vi "uDAQreadData.vi"(4 "Data Header":u8[](array[numeric])=[0, 255, 0], 5 "Process":string, 6 "DataStart":i32, 7 "Residual Buffer in":string[](array[string])=["", "", "", "", "", "", "", ""], 9 "ByteArray":u8[](array[numeric])=array[5000 elements], 10 "FS Range":sgl, 11 "NextArrayBuf":i32) -> (1 "Data":dbl[](array[numeric]), 3 "Residual Buffer out":string[](array[string]))   [LabVIEW 2017]
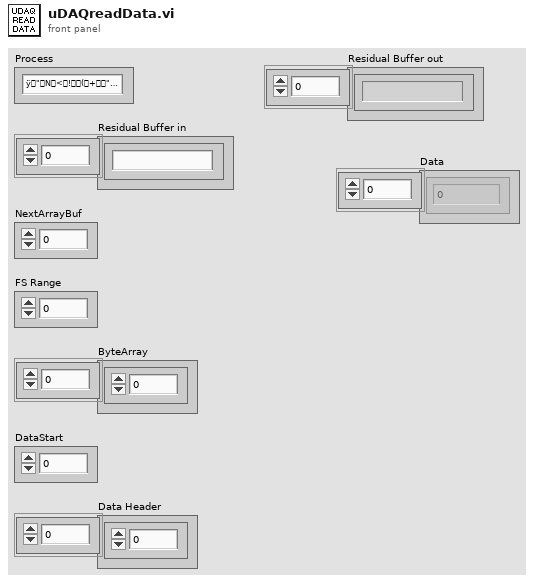
[diagram p1: front panel]
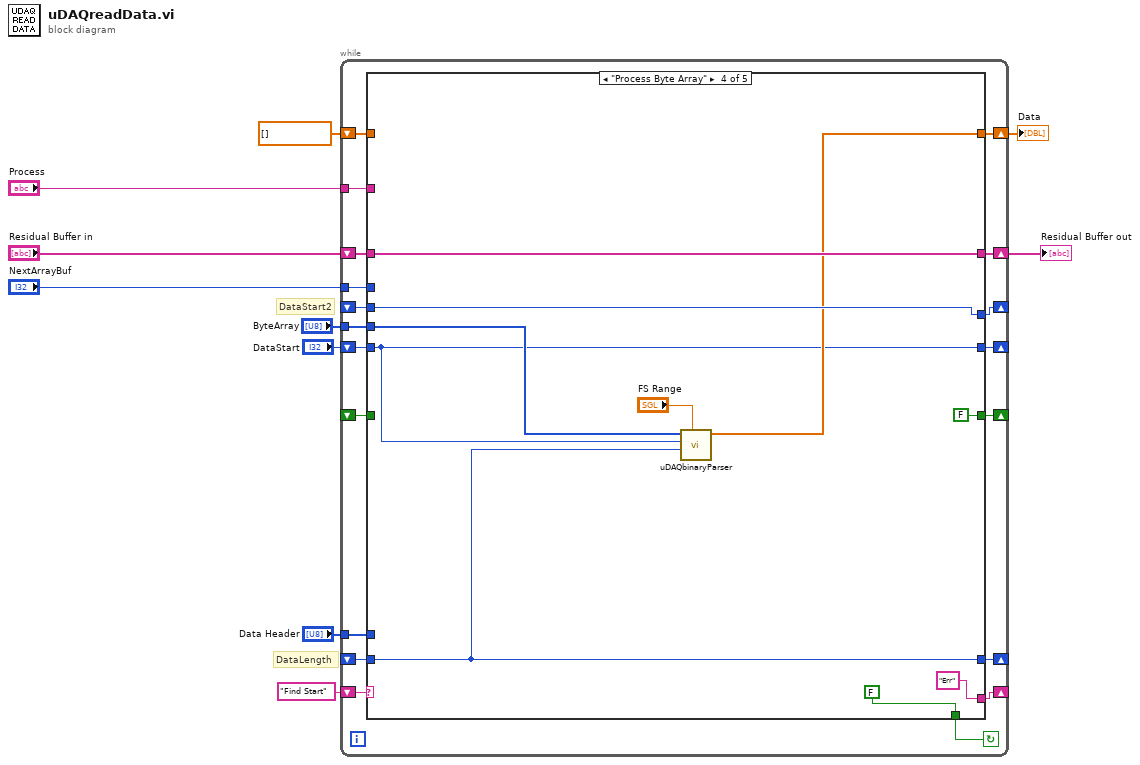
[diagram p0: block diagram]
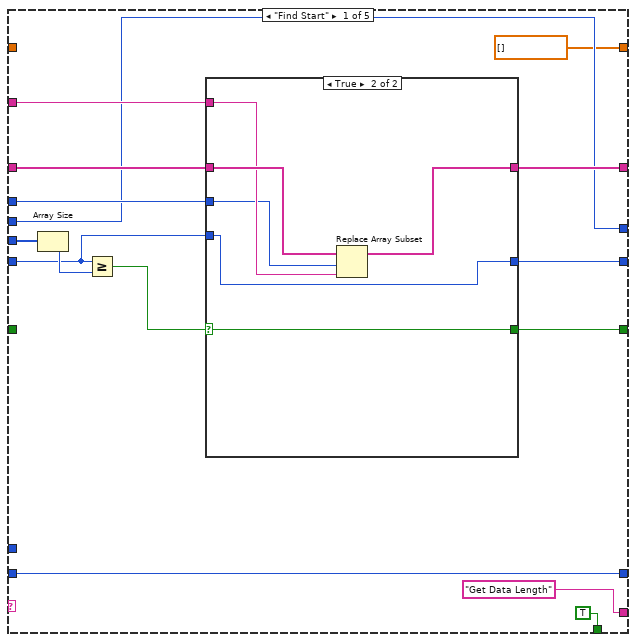
[diagram p2: hidden frame]
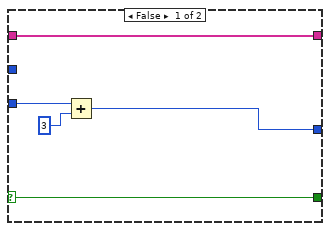
[diagram p3: hidden frame]
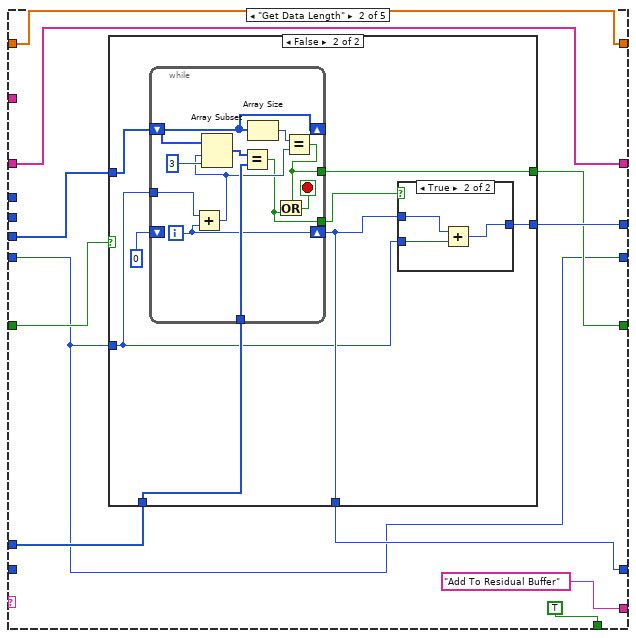
[diagram p4: hidden frame]
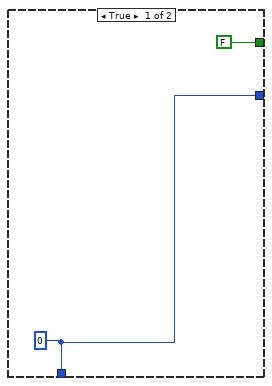
[diagram p5: hidden frame]
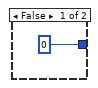
[diagram p6: hidden frame]
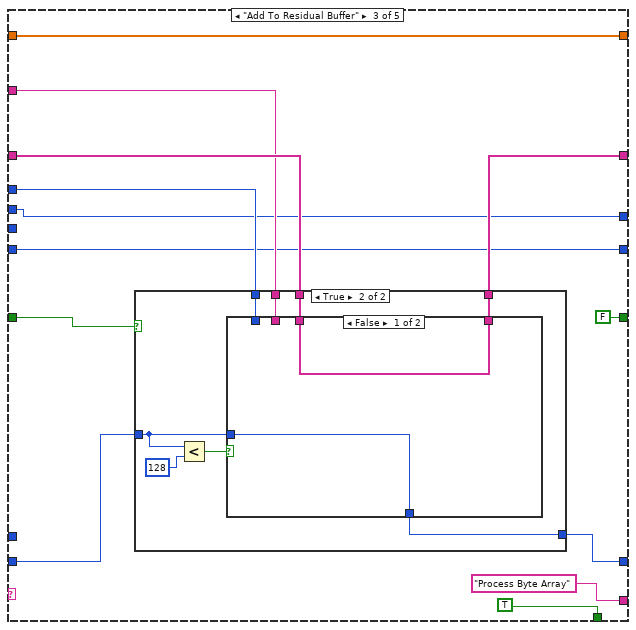
[diagram p7: hidden frame]
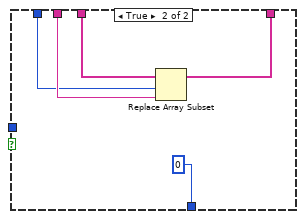
[diagram p9: hidden frame]
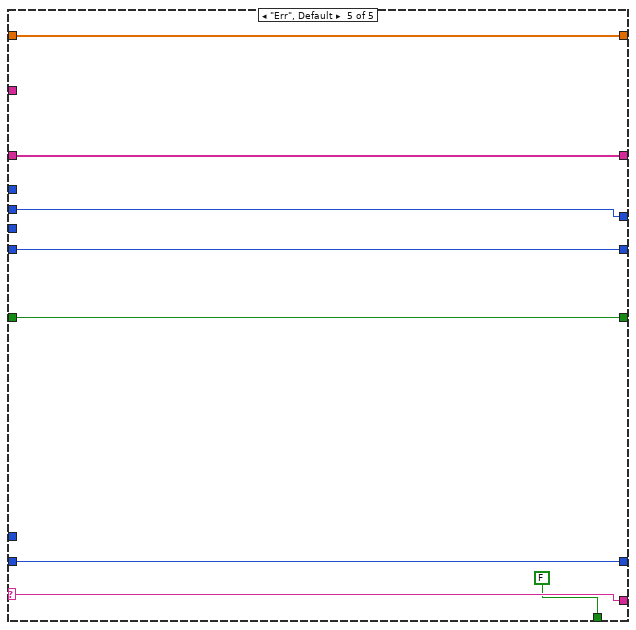
[diagram p10: hidden frame]
diagram:
  # "DataLength"
  # "DataStart2"
  n1 = while {
    shift-right: [w28] -> _
    shift-left: "Find Start" -> [w29]
    tunnel: "Data Header" -> [w25]
    shift-right: [w23] -> w8
    shift-left: "Residual Buffer in" -> [w24]
    tunnel: "Process" -> [w22]
    tunnel: "NextArrayBuf" -> [w21]
    shift-right: [w19] -> _
    shift-left: _ -> [w18]
    shift-right: [w17] -> _
    shift-left: _ -> [w16]
    shift-right: [w14] -> _
    shift-left: _ -> [w15]
    tunnel: "ByteArray" -> [w26]
    shift-right: [w13] -> w1
    shift-left: cdb[] [] ("Data") -> [w12]
    shift-right: [w11] -> _
    shift-left: "DataStart" -> [w27]
    stop <- w20 continue-if-true
    n2 = case shown="\"Process Byte Array\"" w29 {
      selector: w29 -> [_ _ _ _ w139]
      tunnel: ["Get Data Length" "Add To Residual Buffer" "Process Byte Array" "Err" w139] -> w28
      tunnel: w27 -> [w38 w56 w92 w122 w132]
      tunnel: w26 -> [w33 w60 _ w131 _]
      tunnel: w25 -> [_ w66 _ _ _]
      tunnel: w24 -> [w42 w59 w101 w127 w134]
      tunnel: [w41 w59 w98 w127 w134] -> w23
      tunnel: w22 -> [w40 _ w100 _ _]
      tunnel: w21 -> [w39 _ w99 _ _]
      tunnel: [TRUE TRUE TRUE FALSE FALSE] -> w20
      tunnel: [w35 w63 FALSE FALSE w136] -> w19
      tunnel: w18 -> [_ w65 w103 _ w136]
      tunnel: [w34 w64 w96 w128 w135] -> w17
      tunnel: w16 -> [w34 _ w96 w128 w135]
      tunnel: w15 -> [w32 _ w102 w125 w137]
      tunnel: [w32 w58 w97 w125 w137] -> w14
      tunnel: [cdb[] [] ("Data") w57 w93 w126 w133] -> w13
      tunnel: w12 -> [_ w57 w93 _ w133]
      tunnel: [w30 w56 w92 w122 w132] -> w11
      frame "Find Start" {
        n3 = Array Size(array=w33) -> (size(s)=w44:i32)
        n4 = Greater Or Equal?(x=w38, y=w44) -> (x >= y?=w43:bool)
        n5 = case shown="True" w43 {
          selector: w43 -> [w45 w50]
          tunnel: w42 -> [w46 w55]
          tunnel: [w46 w54] -> w41
          tunnel: w40 -> [_ w53]
          tunnel: w39 -> [_ w52]
          tunnel: w38 -> [w49 w51]
          tunnel: [w47 w51] -> w30
          tunnel: [w45 w50] -> w35
          frame False {
            n6 = Add(x=w49, y=3) -> (x+y=w47:i32)
          }
          frame True {
            n7 = Replace Array Subset(array=w55, new element=w53, index=w52) -> (w54:string[])
          }
        }
      }
      frame "Get Data Length" {
        n8 = case shown="False" w65 {
          tunnel: w66 -> [_ w76]
          tunnel: w60 -> [_ w75]
          tunnel: [w67 w71] -> w58
          tunnel: [FALSE w74] -> w63
          tunnel: w56 -> [_ w69]
          tunnel: [w67 w70] -> w64
          frame True {
            w67 = 0
          }
          frame False {
            n9 = while {
              tunnel: w76 -> [w88]
              shift-right: [w85] -> w71
              shift-left: 0 -> [_]
              tunnel: [w84] -> w74
              shift-right: [w83] -> _
              shift-left: w75 -> [w83]
              tunnel: [w82] -> w72
              tunnel: w69 -> [w81]
              i -> [w85]
              stop <- w89 stop-if-true
              n10 = Add(x=w81, y=w85) -> (x+y=w86:i32)
              n11 = Array Subset(array=w83, index=w86, length=3) -> (w90:u8[])
              n12 = Equal?(x=w90, y=w88) -> (x = y?=w82:bool)
              n13 = Array Size(array=w83) -> (size(s)=w87:i32)
              n14 = Equal?(x=w87, y=w86) -> (x = y?=w84:bool)
              n15 = Or(x=w84, y=w82) -> (x .or. y?=w89:bool)
            }
            n16 = case shown="True" w72 {
              tunnel: w71 -> [_ w80]
              tunnel: [0 w79] -> w70
              tunnel: w69 -> [_ w78]
              frame False {
              }
              frame True {
                n17 = Add(x=w80, y=w78) -> (x+y=w79:i32)
              }
            }
          }
        }
      }
      frame "Add To Residual Buffer" {
        n18 = case shown="True" w103 {
          tunnel: w102 -> [w106 w107]
          tunnel: w101 -> [w105 w112]
          tunnel: w100 -> [_ w111]
          tunnel: w99 -> [_ w110]
          tunnel: [w105 w109] -> w98
          tunnel: [w106 w108] -> w97
          frame False {
          }
          frame True {
            n19 = Less?(x=w107, y=u8 128 ("number")) -> (x < y?=w113:bool)
            n20 = case shown="False" w113 {
              tunnel: w112 -> [w115 w121]
              tunnel: w111 -> [_ w120]
              tunnel: w110 -> [_ w119]
              tunnel: [w115 w118] -> w109
              tunnel: [w116 0] -> w108
              tunnel: w107 -> [w116 _]
              frame False {
              }
              frame True {
                n21 = Replace Array Subset(array=w121, new element=w120, index=w119) -> (w118:string[])
              }
            }
          }
        }
      }
      frame "Process Byte Array" {
        n22 = call "uDAQbinaryParser.vi"("FS Range"="FS Range", "DataLength"=w125, "DataStart"=w122, "ByteArray"=w131) -> ("Data"=w126:dbl[])  [unwired: 7 in]
      }
      frame "Err", Default {
      }
    }
  }
  "Residual Buffer out" <- w8
  "Data" <- w1
